vi "Calibrate Camera.vi"(0 "Image In":T1, 5 "Image Dst":T1, 7 "File Path (Image Calibration 1)":path=path "C:/Users/wobot/OneDrive/Desktop/Calibrations/Dots/Cam2.png", 11 "error in":errorcluster) -> (4 "Image Out":T1, 8 "Execution Time":u32)   [LabVIEW 2023]
doc: "Creates, edits, and runs vision algorithms using NI Vision Assistant.\n\nWhen you place this Express VI on the block diagram, NI Vision Assistant launches. Create an algorithm using the Vision Assistant processing functions. After you create an algorithm, you can select the controls and indicators that you want to be able to programmatically set in LabVIEW. Double-click the Vision Assistant Express VI to edit the algorithm."
uses:
  <vilib>/vision/Image Controls.llb/IMAQ Image.ctl
  <vilib>/vision/NI_Vision_Development_Module.lvlib
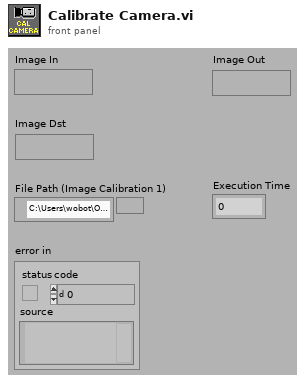
[diagram p1: front panel]
types:
  T1 = typedef "IMAQ Image.ctl" = refnum<image>
  T2 = cluster{"Origin Pixel":cluster{"X":sgl, "Y":sgl}, "X Axis Pixel":cluster{"X":sgl, "Y":sgl}, "Axis Reference":u32}
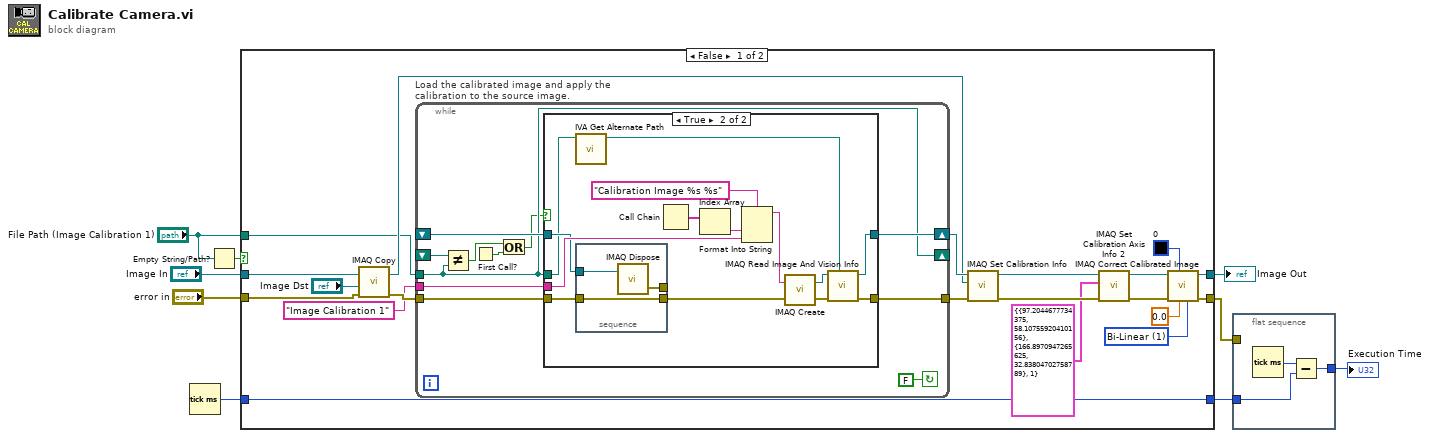
[diagram p0: block diagram]
diagram:
  n1 = Tick Count (ms)() -> (millisecond timer value=w4:u32)
  n2 = Empty String/Path?(string/path="File Path (Image Calibration 1)") -> (empty?=w6:bool)
  n3 = case shown="False" w6 {
    tunnel: "Image In" -> [w28 w61]
    tunnel: [w17 _] -> w3
    tunnel: [w13 w61] -> w8
    tunnel: "File Path (Image Calibration 1)" -> [w12 _]
    tunnel: "error in" -> [w11 _]
    tunnel: w4 -> [w10 w60]
    tunnel: [w10 w60] -> w2
    frame False {
      w18 = u32 1 items=["Zero Order", "Bi-Linear", "Quadratic", "Cubic Spline"] ("Interpolation Type")
      n4 = call "IMAQ Copy"("error in (no error)"=w11, "Image Dst"="Image Dst", "Image Src"=w28) -> ("error out"=w27:errorcluster, "Image Dst Out"=w23:T1)  [unwired: 3 out]
      n5 = while "Load the calibrated image and apply the calibration to the source image." {
        shift-right: [w40] -> w26
        shift-left: _ -> [w39]
        tunnel: [w37] -> w25
        tunnel: w27 -> [w36]
        tunnel: w12 -> [w33]
        tunnel: "Image Calibration 1" ("Step Name") -> [w35]
        shift-right: [w33] -> _
        shift-left: _ -> [w34]
        stop <- FALSE continue-if-true
        n6 = Not Equal?(x=w34, y=w33) -> (x != y?=w31:bool)
        n7 = First Call?() -> (First Call?: T/F=w32:bool)
        n8 = Or(x=w31, y=w32) -> (x .or. y?=w30:bool)
        n9 = case shown="True" w30 {
          tunnel: [w42 w54] -> w40
          tunnel: w39 -> [w42 w46]
          tunnel: [w41 w51] -> w37
          tunnel: w36 -> [w41 w47]
          tunnel: w33 -> [_ w44]
          tunnel: w35 -> [_ w48]
          frame False {
          }
          frame True {
            n10 = call <vilib>:"IVA Get Alternate Path.vi"("Path In"=w44) -> ("Path Out"=w43:path)  [unwired: 10 out]
            n11 = stacked-sequence {
              tunnel: w47 -> [w58]
              tunnel: w46 -> [w59]
              tunnel: [w58] -> w45
              tunnel: [w57] -> _
              frame #0 {
                n12 = call "IMAQ Dispose"("Image"=w59) -> ("error out"=w57:errorcluster)  [unwired: 2 in, 3 out]
              }
            }
            n13 = Call Chain() -> (call chain=w50:string[])
            n14 = Index Array(array=w50) -> (element=w49:string)  [unwired: 1 in]
            n15 = Format Into String(format string="Calibration Image %s %s" ("Image Name"), w49, w48) -> (resulting string=w56:string)  [unwired: 2 in, 1 out]
            n16 = call "IMAQ Create"("Image Name"=w56, "error in (no error)"=w45) -> ("New Image"=w53:T1, "error out"=w52:errorcluster)  [unwired: 2 in, 1 out]
            n17 = call "IMAQ Read Image And Vision Info"("File Path"=w43, "error in (no error)"=w52, "Image"=w53) -> ("error out"=w51:errorcluster, "Image Out"=w54:T1)  [unwired: 1 in, 6 out]
          }
        }
      }
      n18 = call "IMAQ Set Calibration Info"("error in (no error)"=w25, "Image Dst"=w23, "Image Src"=w26) -> ("error out"=w24:errorcluster, "Calibrated Image"=w20:T1)  [unwired: 1 in, 6 out]
      n19 = call-poly "IMAQ Set Calibration Axis Info 2"("error in (no error)"=w24, "Calibration Axis Info"=T2 {"Origin Pixel"={"X"=97.20447, "Y"=58.10756}, "X Axis Pixel"={"X"=166.8971, "Y"=32.838047}, "Axis Reference"=1}, "Calibration Template Image In"=w20) -> ("error out"=w21:errorcluster, "Calibration Template Image Out"=w16:T1)  [unwired: 7 out]
      n20 = call "IMAQ Correct Calibrated Image"("Interpolation Type"=w18, "Replace Value"=sgl 0.0, "Color Replace Value"=u32 0, "error in (no error)"=w21, "Image Src"=w16) -> ("error out"=w17:errorcluster, "Corrected Image"=w13:T1)  [unwired: 2 in, 3 out]
    }
    frame True {
    }
  }
  "Image Out" <- w8
  n21 = flat-sequence {
    tunnel: w3 -> [_]
    tunnel: w2 -> [w63]
    tunnel: [w62] -> w1
    frame #0 {
      n22 = Tick Count (ms)() -> (millisecond timer value=w64:u32)
      n23 = Subtract(x=w64, y=w63) -> (x-y=w62:u32)
    }
  }
  "Execution Time" <- w1
